vi "Intensity_png.vi"(3 "No of Contours":i32=20, 4 "Job Directory":path=path "/Lacie_20/paulhayden/Documents/EnFlo bits/EnFlo Tun Vel profiles/View_LDA data.tpt", 5 "Intensity Graph":dbl[][](graph)) -> ()   [LabVIEW 2010]
uses:
  Results_plotter_Global.vi
panel:
  out "String":string
  in  "Added labels":i32[](listbox)
  in  "Z Min":dbl=0.97
  in  "Z Max":dbl=1.07
  in  "Save Automatically?":bool
  in  "Auto scale Intensity":bool=TRUE
  in  "Colour":bool=TRUE
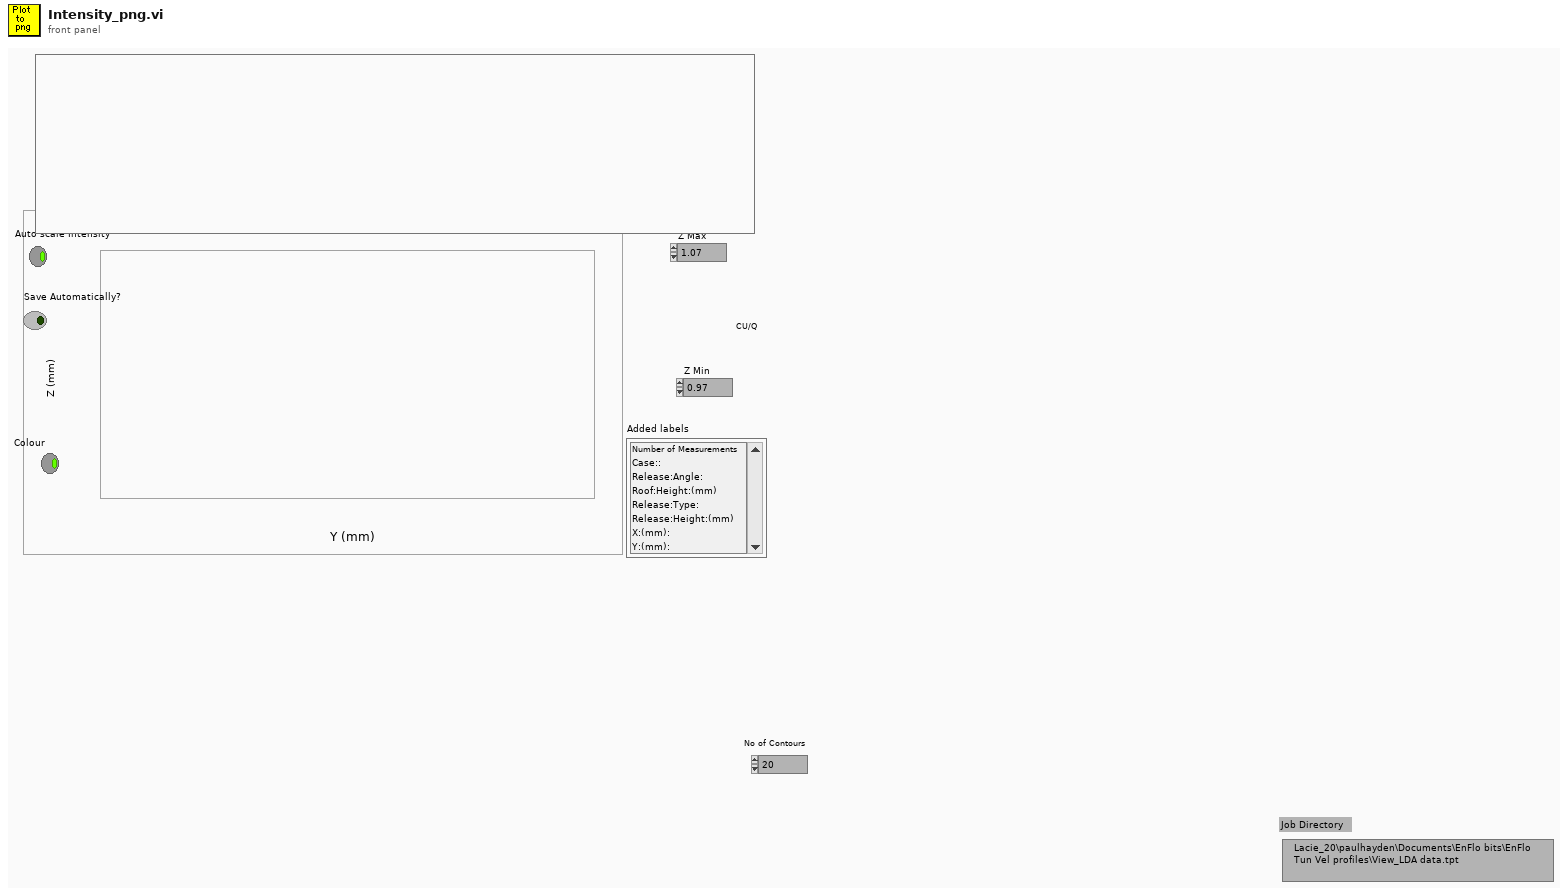
[diagram p1: front panel]
types:
  T1 = typedef "LVRectTypeDef.ctl" = cluster{"left":i16, "top":i16, "right":i16, "bottom":i16}
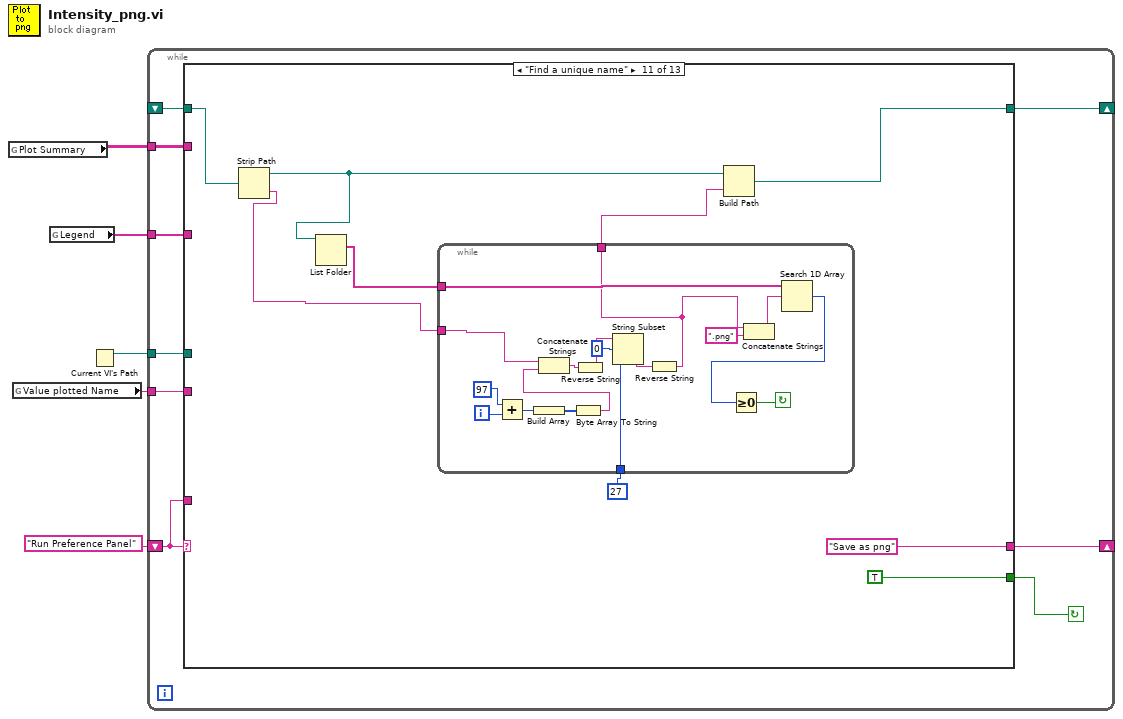
[diagram p0: block diagram]
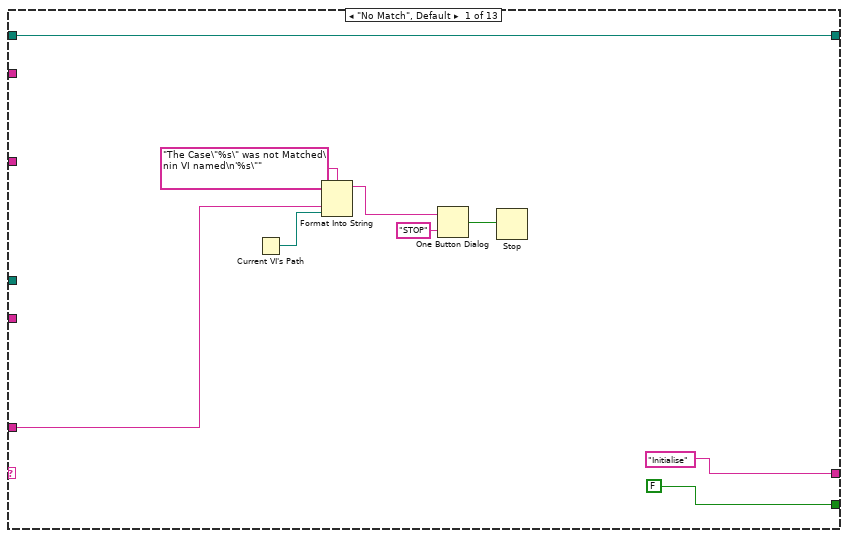
[diagram p2: hidden frame]
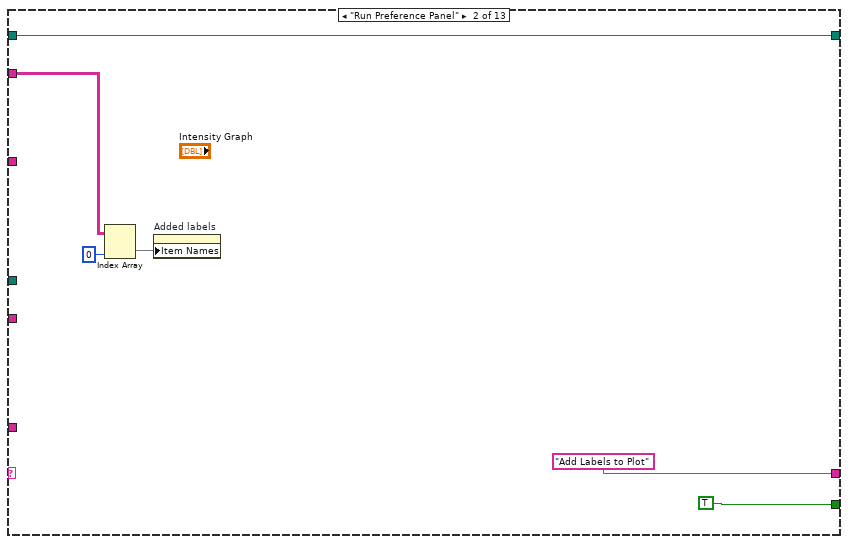
[diagram p3: hidden frame]
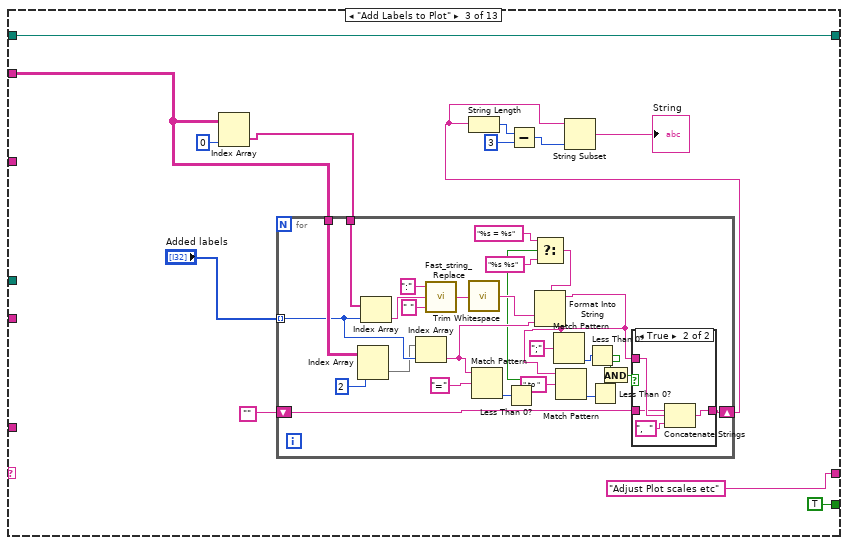
[diagram p4: hidden frame]
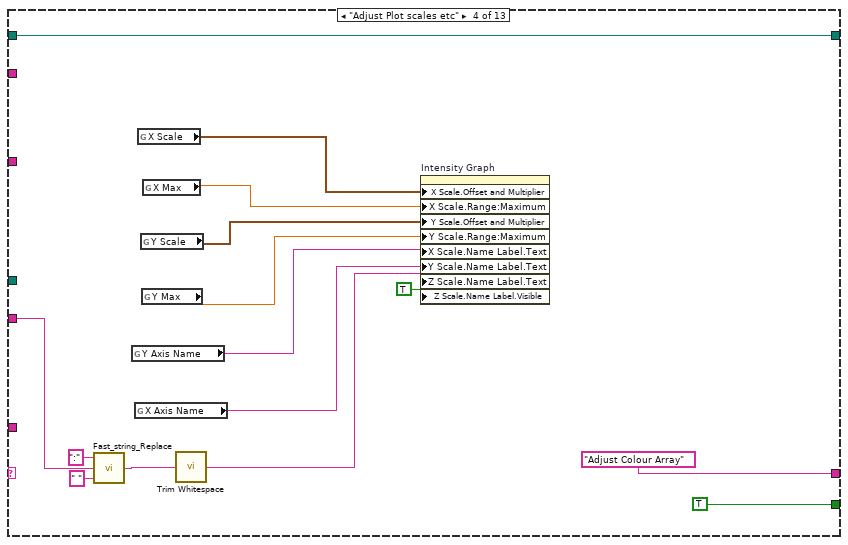
[diagram p6: hidden frame]
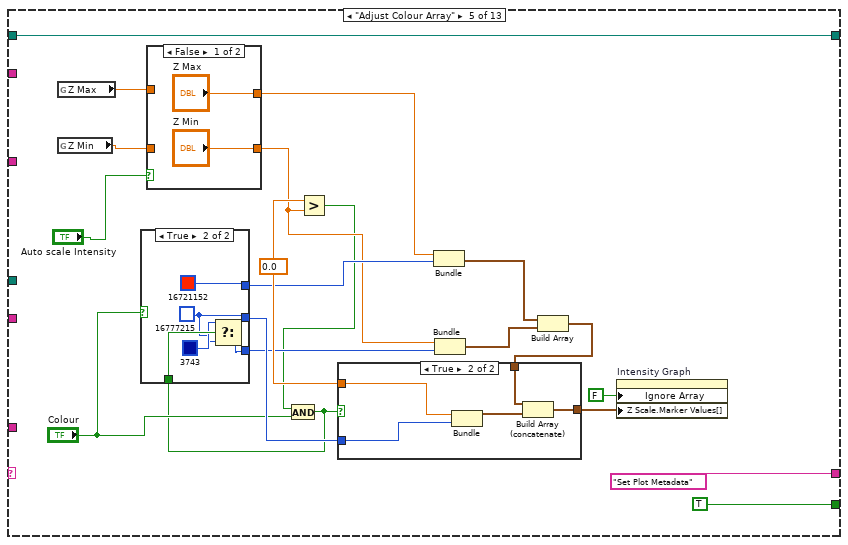
[diagram p7: hidden frame]
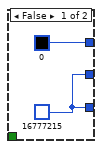
[diagram p8: hidden frame]
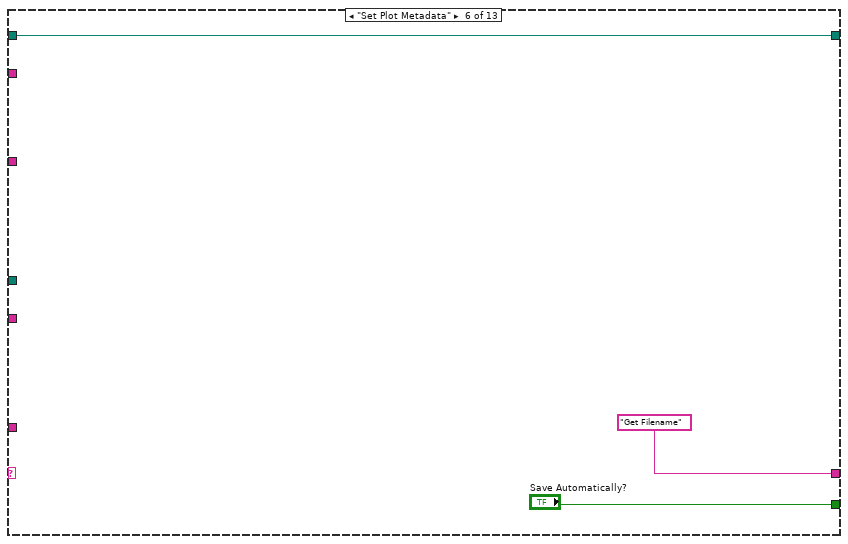
[diagram p11: hidden frame]
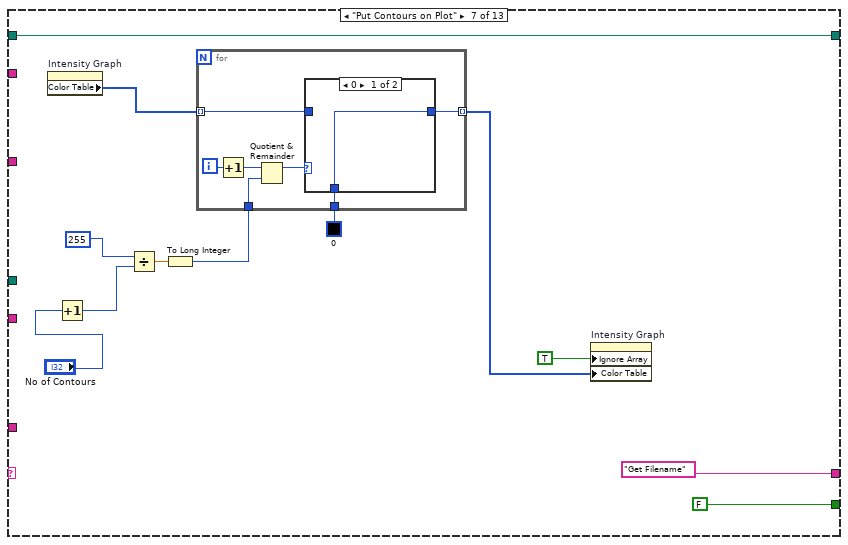
[diagram p12: hidden frame]
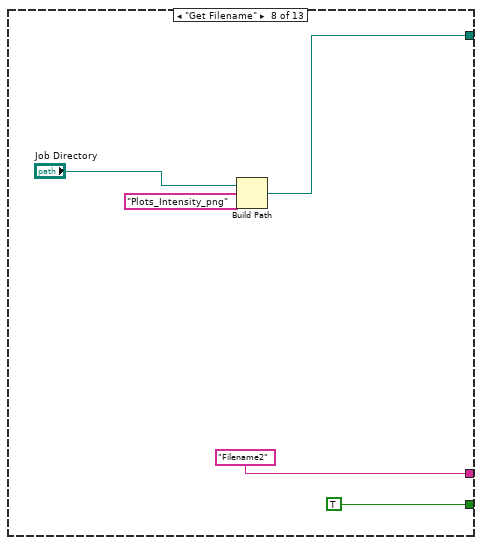
[diagram p14: hidden frame]
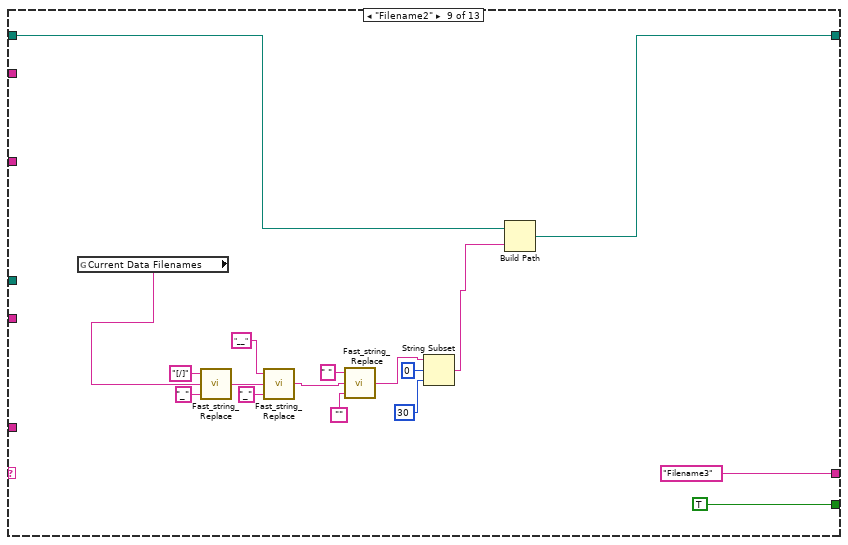
[diagram p15: hidden frame]
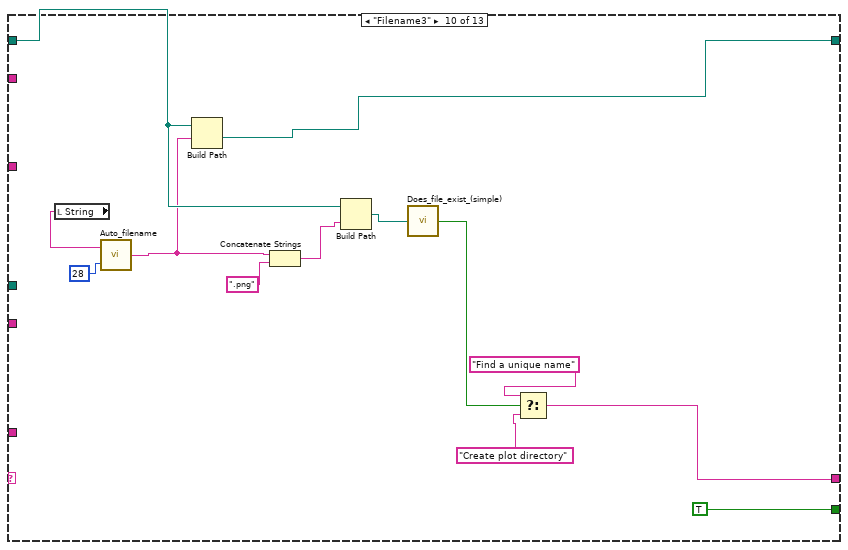
[diagram p16: hidden frame]
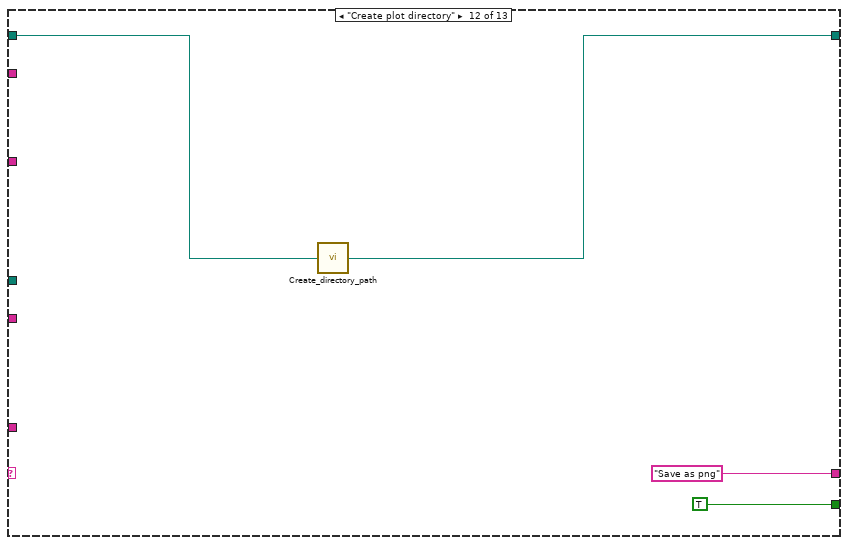
[diagram p17: hidden frame]
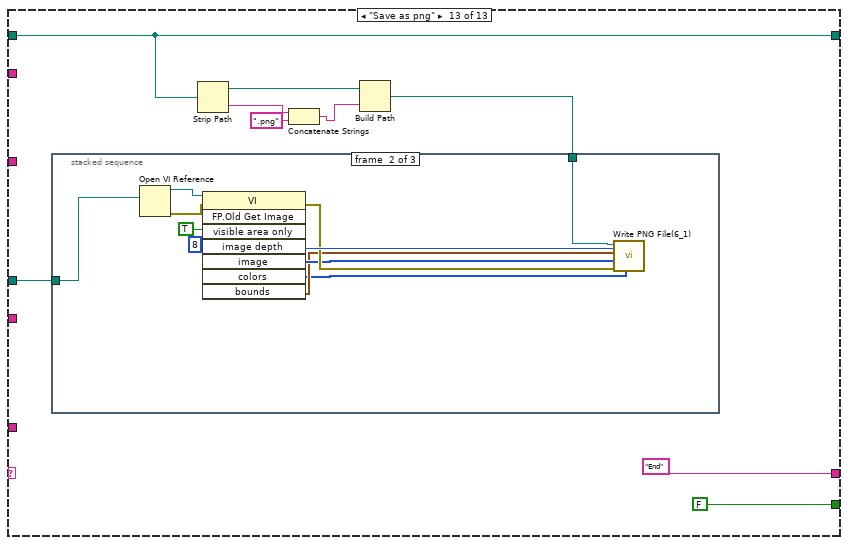
[diagram p18: hidden frame]
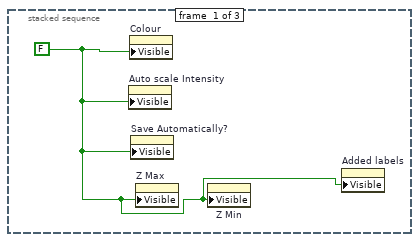
[diagram p19: hidden frame]
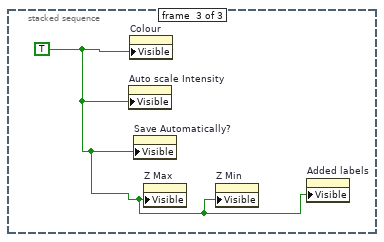
[diagram p20: hidden frame]
diagram:
  n1 = global read "Results_plotter_Global.vi" "Plot Summary"() -> (w1:string[][])
  n2 = global read "Results_plotter_Global.vi" "Value plotted Name"() -> (w3:string)
  n3 = global read "Results_plotter_Global.vi" "Legend"() -> (w2:string[])
  n4 = Current VI's Path() -> (path=w4:path)
  n5 = while {
    shift-left: "Run Preference Panel" -> [w12]
    shift-right: [w13] -> _
    tunnel: w4 -> [w11]
    shift-right: [w10] -> _
    shift-left: _ -> [w9]
    tunnel: w3 -> [w8]
    tunnel: w2 -> [w7]
    tunnel: w1 -> [w6]
    stop <- w14 continue-if-true
    n6 = case shown="\"Find a unique name\"" w12 {
      tunnel: [FALSE TRUE TRUE ("Top Level") TRUE ("Top Level") TRUE ("Top Level") "Save Automatically?" FALSE ("Top Level") TRUE ("Top Level") TRUE ("Top Level") TRUE ("Top Level") TRUE ("Top Level") TRUE ("Top Level") FALSE ("Top Level")] -> w14
      tunnel: ["Initialise" "Add Labels to Plot" "Adjust Plot scales etc" "Adjust Colour Array" "Set Plot Metadata" "Get Filename" "Get Filename" "Filename2" "Filename3" w182 "Save as png" "Save as png" "End"] -> w13
      tunnel: w12 -> [w18 _ _ _ _ _ _ _ _ _ _ _ _]
      tunnel: w11 -> [_ _ _ _ _ _ _ _ _ _ _ _ w223]
      tunnel: [w15 w27 w38 w80 w98 w128 w130 w153 w158 w183 w188 w212 w220] -> w10
      tunnel: w9 -> [w15 w27 w38 w80 w98 w128 w130 _ w159 w184 w189 w213 w220]
      tunnel: w8 -> [_ _ _ w79 _ _ _ _ _ _ _ _ _]
      tunnel: w7 -> [_ _ _ _ _ _ _ _ _ _ _ _ _]
      tunnel: w6 -> [_ w25 w42 _ _ _ _ _ _ _ _ _ _]
      frame "No Match", Default {
        n7 = Current VI's Path() -> (path=w17:path)
        n8 = Format Into String(format string="The Case\"%s\" was not Matched\nin VI named\n'%s\"" ("Format String"), w18, w17) -> (resulting string=w21:string)  [unwired: 2 in, 1 out]
        n9 = One Button Dialog(message=w21, button name ("OK")="STOP") -> (true=w19:bool)
        n10 = Stop(stop? (T)=w19) -> ()
      }
      frame "Run Preference Panel" {
        n11 = Index Array(array=w25, index (col)=0 ("disabled index (col)")) -> (element=w24:string[])  [unwired: 1 in]
        n12 = property on="Added labels" class="LstBox (strict)"("Item Names"=w24) -> ()  [unwired: 2 in, 2 out]
      }
      frame "Add Labels to Plot" {
        n13 = Index Array(array=w42, index (col)=0 ("disabled index (col)")) -> (element=w40:string[])  [unwired: 1 in]
        n14 = for {
          tunnel: "Added labels" -> [w67] mode=indexing
          tunnel: w40 -> [w69]
          tunnel: w42 -> [w68]
          shift-right: [w58] -> w31
          shift-left: "" -> [w59]
          n15 = Index Array(array=w68, index (col)=2 ("disabled index (col)")) -> (element=w66:string[])  [unwired: 1 in]
          n16 = Index Array(array=w69, index=w67) -> (element=w63:string)
          n17 = Index Array(array=w66, index=w67) -> (element=w57:string)
          n18 = call "Fast_string_Replace.vi"("Replace match with:"=" ", "Input String"=w63, "regular expression"=":") -> ("Output String"=w62:string)  [unwired: 2 out]
          n19 = call <vilib>:"Trim Whitespace.vi"("string"=w62) -> ("trimmed string"=w61:string)  [unwired: 1 in]
          n20 = Match Pattern(string=w57, regular expression="=") -> (offset past match=w55:i32)  [unwired: 4 out]
          n21 = Less Than 0?(x=w55) -> (x < 0?=w54:bool)
          n22 = Select(t="%s = %s" ("format string"), s=w54, f="%s %s" ("format string")) -> (s? t:f=w51:string)
          n23 = Format Into String(format string=w51, w61, w57) -> (resulting string=w44:string)  [unwired: 2 in, 1 out]
          n24 = Match Pattern(string=w44, regular expression=";") -> (offset past match=w49:i32)  [unwired: 4 out]
          n25 = Match Pattern(string=w44, regular expression=" to ") -> (offset past match=w48:i32)  [unwired: 4 out]
          n26 = Less Than 0?(x=w49) -> (x < 0?=w46:bool)
          n27 = Less Than 0?(x=w48) -> (x < 0?=w47:bool)
          n28 = And(x=w46, y=w47) -> (x .and. y?=w45:bool)
          n29 = case shown="True" w45 {
            tunnel: w59 -> [w70 w72]
            tunnel: [w70 w73] -> w58
            tunnel: w44 -> [_ w74]
            frame False {
            }
            frame True {
              n30 = Concatenate Strings(w72, w74, ",  " ("string")) -> (w73:string)
            }
          }
        }
        n31 = String Length(string=w31) -> (length=w34:i32)
        n32 = Subtract(x=w34, y=3) -> (x-y=w32:i32)
        n33 = String Subset(string=w31, length (rest)=w32) -> (substring=→"String":string)  [unwired: 1 in]
      }
      frame "Adjust Plot scales etc" {
        n34 = call "Fast_string_Replace.vi"("Replace match with:"=" ", "Input String"=w79, "regular expression"=":") -> ("Output String"=w76:string)  [unwired: 1 in, 1 out]
        n35 = global read "Results_plotter_Global.vi" "Y Axis Name"() -> (w83:string)
        n36 = global read "Results_plotter_Global.vi" "X Axis Name"() -> (w82:string)
        n37 = global read "Results_plotter_Global.vi" "X Scale"() -> (w88:cluster{"Xo":dbl, "delta X":dbl})
        n38 = global read "Results_plotter_Global.vi" "Y Scale"() -> (w86:cluster{"Xo":dbl, "delta X":dbl})
        n39 = global read "Results_plotter_Global.vi" "Y Max"() -> (w85:dbl)
        n40 = global read "Results_plotter_Global.vi" "X Max"() -> (w87:dbl)
        n41 = call <vilib>:"Trim Whitespace.vi"("string"=w76) -> ("trimmed string"=w75:string)  [unwired: 1 in]
        n42 = property on="Intensity Graph" class="IntGraph (strict)"("X Scale.Offset and Multiplier"=w88, "X Scale.Range:Maximum"=w87, "Y Scale.Offset and Multiplier"=w86, "Y Scale.Range:Maximum"=w85, "X Scale.Name Label.Text"=w83, "Y Scale.Name Label.Text"=w82, "Z Scale.Name Label.Text"=w75, "Z Scale.Name Label.Visible"=TRUE) -> ()  [unwired: 2 in, 2 out]
      }
      frame "Adjust Colour Array" {
        w109 = 0.0 ("max Z value")
        n43 = global read "Results_plotter_Global.vi" "Z Max"() -> (w96:dbl)
        n44 = global read "Results_plotter_Global.vi" "Z Min"() -> (w94:dbl)
        n45 = case shown="False" "Auto scale Intensity" {
          tunnel: ["Z Max" w120] -> w97
          tunnel: w96 -> [_ w120]
          tunnel: ["Z Min" w119] -> w95
          tunnel: w94 -> [_ w119]
          frame False {
          }
          frame True {
          }
        }
        n46 = Greater?(x=w109, y=w95) -> (0:w92:bool)
        n47 = And(x=w92, y="Colour") -> (x .and. y?=w90:bool)
        n48 = case shown="True" "Colour" {
          tunnel: [w111 w112] -> w105
          tunnel: [u32 0 u32 16721152] -> w104
          tunnel: [w111 w113] -> w100
          tunnel: w90 -> [_ w115]
          frame False {
            w111 = u32 16777215
          }
          frame True {
            w112 = u32 16777215
            n49 = Select(t=u32 3743, s=w115, f=w112) -> (s? t:f=w113:u32)
          }
        }
        n50 = Bundle("Z Max"=w97, w104) -> (w106:cluster{"Z Max":dbl, u32})  [unwired: 1 in]
        n51 = Bundle("Z Min"=w95, w100) -> (w108:cluster{"Z Min":dbl, u32})  [unwired: 1 in]
        n52 = Build Array(w106, w108) -> (w107:cluster{"Z Min":dbl, u32}[])
        n53 = case shown="True" w90 {
          tunnel: w107 -> [w121 w126]
          tunnel: [w121 w124] -> w102
          tunnel: w105 -> [_ w123]
          tunnel: w109 -> [_ w122]
          frame False {
          }
          frame True {
            n54 = Bundle("max Z value"=w122, w123) -> (w125:cluster{"max Z value":dbl, u32})  [unwired: 1 in]
            n55 = Build Array (concatenate)(w126, w125) -> (w124:cluster{"max Z value":dbl, u32}[])
          }
        }
        n56 = property on="Intensity Graph" class="IntGraph (strict)"("Ignore Array"=FALSE, "Z Scale.Marker Values[]"=w102) -> ()  [unwired: 2 in, 2 out]
      }
      frame "Set Plot Metadata" {
      }
      frame "Put Contours on Plot" {
        n57 = property on="Intensity Graph" class="IntGraph (strict)"() -> ("Color Table"=w133:u32[])  [unwired: 2 in, 2 out]
        n58 = Increment(x="No of Contours") -> (x+1=w138:i32)
        n59 = Divide(x=255, y=w138) -> (x/y=w137:dbl)
        n60 = To Long Integer(number=w137) -> (32bit integer=w135:i32)
        n61 = for {
          tunnel: w135 -> [w147]
          tunnel: [w144] -> w132 mode=indexing
          tunnel: w133 -> [w143] mode=indexing
          tunnel: u32 0 -> [w142]
          i -> [w148]
          n62 = Increment(x=w148) -> (x+1=w145:i32)
          n63 = Quotient & Remainder(x=w145, y=w147) -> (x-y*floor(x/y)=w146:i32)  [unwired: 1 out]
          n64 = case shown="0" w146 {
            tunnel: [w149 w150] -> w144
            tunnel: w143 -> [_ w150]
            tunnel: w142 -> [w149 _]
            frame 0 {
            }
            frame 1, Default {
            }
          }
        }
        n65 = property on="Intensity Graph" class="IntGraph (strict)"("Ignore Array"=TRUE, "Color Table"=w132) -> ()  [unwired: 2 in, 2 out]
      }
      frame "Get Filename" {
        n66 = Build Path(base path="Job Directory", name or relative path="Plots_Intensity_png") -> (appended path=w153:path)
      }
      frame "Filename2" {
        n67 = global read "Results_plotter_Global.vi" "Current Data Filenames"() -> (w170:string)
        n68 = call "Fast_string_Replace.vi"("Replace match with:"="_", "Input String"=w170, "regular expression"="[/]") -> ("Output String"=w166:string)  [unwired: 1 in, 1 out]
        n69 = call "Fast_string_Replace.vi"("Replace match with:"="_", "Input String"=w166, "regular expression"="__") -> ("Output String"=w169:string)  [unwired: 1 in, 1 out]
        n70 = call "Fast_string_Replace.vi"("Replace match with:"="", "Input String"=w169, "regular expression"=" ") -> ("Output String"=w171:string)  [unwired: 1 in, 1 out]
        n71 = String Subset(string=w171, offset (0)=0, length (rest)=30 ("length (rest)")) -> (substring=w172:string)
        n72 = Build Path(base path=w159, name or relative path=w172) -> (appended path=w158:path)
      }
      frame "Filename3" {
        n73 = local read "String"() -> (w173:string)
        n74 = call "Auto_filename.vi"("Filename Max length"=28, "Prefix"=w173) -> ("Filename"=w175:string)
        n75 = Build Path(base path=w184, name or relative path=w175) -> (appended path=w183:path)
        n76 = Concatenate Strings(w175, ".png" ("string")) -> (w180:string)
        n77 = Build Path(base path=w184, name or relative path=w180) -> (appended path=w179:path)
        n78 = call "Does_file_exist_(simple).vi"("Pathname"=w179) -> ("exists?"=w178:bool)
        n79 = Select(t="Find a unique name", s=w178, f="Create plot directory") -> (s? t:f=w182:string)
      }
      frame "Find a unique name" {
        n80 = Strip Path(path=w189) -> (stripped path=w187:path, name=w191:string)
        n81 = List Folder(path=w187) -> (filenames=w186:string[])  [unwired: 3 in, 3 out]
        n82 = while {
          tunnel: w191 -> [w211]
          tunnel: 27 ("Max Length") -> [w210]
          tunnel: [w196] -> w192
          tunnel: w186 -> [w200]
          i -> [w201]
          stop <- w198 continue-if-true
          n83 = Add(x=97, y=w201) -> (x+y=w208:i32)
          n84 = Build Array(w208) -> (w209:i32[])
          n85 = Byte Array To String(unsigned byte array=w209) -> (string=w206:string)
          n86 = Concatenate Strings(w211, w206) -> (w204:string)
          n87 = Reverse String(1:w204) -> (0:w205:string)
          n88 = String Subset(string=w205, offset (0)=0, length (rest)=w210) -> (substring=w203:string)
          n89 = Reverse String(1:w203) -> (0:w196:string)
          n90 = Concatenate Strings(w196, ".png" ("string")) -> (w195:string)
          n91 = Search 1D Array(1D array=w200, element=w195) -> (index of element=w199:i32)  [unwired: 1 in]
          n92 = Greater Or Equal To 0?(x=w199) -> (x >= 0?=w198:bool)
        }
        n93 = Build Path(base path=w187, name or relative path=w192) -> (appended path=w188:path)
      }
      frame "Create plot directory" {
        n94 = call "Create_directory_path.vi"("Path name"=w213) -> ("Path name Out"=w212:path)
      }
      frame "Save as png" {
        n95 = Strip Path(path=w220) -> (stripped path=w221:path, name=w219:string)
        n96 = Concatenate Strings(w219, ".png" ("string")) -> (w218:string)
        n97 = Build Path(base path=w221, name or relative path=w218) -> (appended path=w216:path)
        n98 = stacked-sequence {
          tunnel: w223 -> [_ w233 _]
          tunnel: w216 -> [_ w226 _]
          frame #0 {
            w225 = FALSE ("Visible")
            n99 = property on="Auto scale Intensity" class="Bool (strict)"("Visible"=w225) -> ()  [unwired: 2 in, 2 out]
            n100 = property on="Colour" class="Bool (strict)"("Visible"=w225) -> ()  [unwired: 2 in, 2 out]
            n101 = property on="Save Automatically?" class="Bool (strict)"("Visible"=w225) -> ()  [unwired: 2 in, 2 out]
            n102 = property on="Z Max" class="DigNum (strict)"("Visible"=w225) -> ()  [unwired: 2 in, 2 out]
            n103 = property on="Z Min" class="DigNum (strict)"("Visible"=w225) -> ()  [unwired: 2 in, 2 out]
            n104 = property on="Added labels" class="LstBox (strict)"("Visible"=w225) -> ()  [unwired: 2 in, 2 out]
          }
          frame #1 {
            w231 = 8 ("image depth")
            n105 = Open VI Reference(vi path=w233) -> (vi reference=w235:refnum<vi>, error out=w234:errorcluster)  [unwired: 5 in]
            n106 = invoke class="VI" method="FP.Old Get Image"(reference=w235, error in=w234, "visible area only"=TRUE, "image depth"=w231) -> (error out=w230:errorcluster, "image"=w229:u8[], "colors"=w227:u32[], "bounds"=w228:T1)  [unwired: 4 in, 4 out]
            n107 = call <vilib>:"Write PNG File(6_1).vi"("color table"=w227, "depth"=w231, "error in (no error)"=w230, "flattened image data"=w229, "rect"=w228, "path to PNG file"=w226) -> ()  [unwired: 4 in, 2 out]
          }
          frame #2 {
            w236 = TRUE ("Visible")
            n108 = property on="Auto scale Intensity" class="Bool (strict)"("Visible"=w236) -> ()  [unwired: 2 in, 2 out]
            n109 = property on="Colour" class="Bool (strict)"("Visible"=w236) -> ()  [unwired: 2 in, 2 out]
            n110 = property on="Save Automatically?" class="Bool (strict)"("Visible"=w236) -> ()  [unwired: 2 in, 2 out]
            n111 = property on="Z Max" class="DigNum (strict)"("Visible"=w236) -> ()  [unwired: 2 in, 2 out]
            n112 = property on="Z Min" class="DigNum (strict)"("Visible"=w236) -> ()  [unwired: 2 in, 2 out]
            n113 = property on="Added labels" class="LstBox (strict)"("Visible"=w236) -> ()  [unwired: 2 in, 2 out]
          }
        }
      }
    }
  }
